vi "comm wait for character.vi"(5 "Loop Delay (10)":u32=10, 7 "timeout (10000)":u32=10000, 8 "error in (no error)":errorcluster, 9 "string in (\"\")":string, 10 "character":string, 11 "Comm Handle":u64) -> (0 "error out":errorcluster, 1 "received data":string, 2 "match":bool, 3 "dup Comm Handle":u64, 4 "before match":string, 6 "after match":string)   [LabVIEW 2021, in "lvserial.lvlib"]
doc: "This VI is receiving the data from the device and searches for the 'character'. If the character matches, the VI returns 'match'=TRUE.\nAfter 'timeout' the 'match' is FALSE and all received data are lost.\n\nThe VI receives only one byte at a time, so all data after the character remain in the serial I/O buffer."
uses:
  lvserial.lvlib
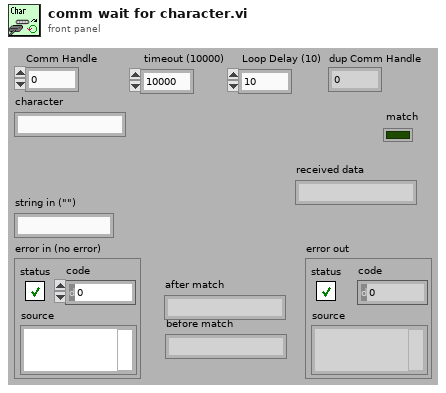
[diagram p1: front panel]
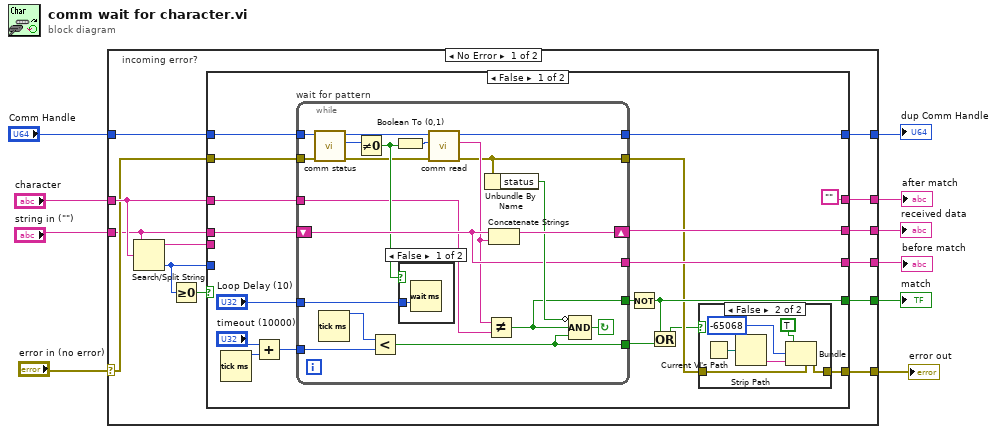
[diagram p0: block diagram]
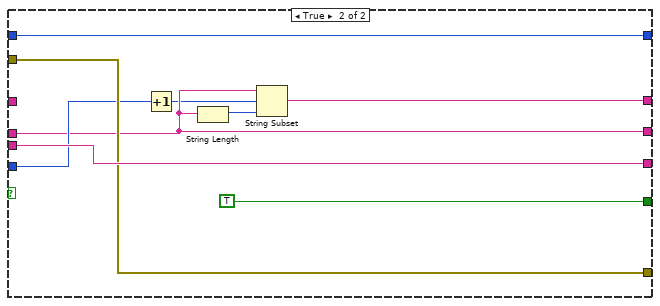
[diagram p4: hidden frame]
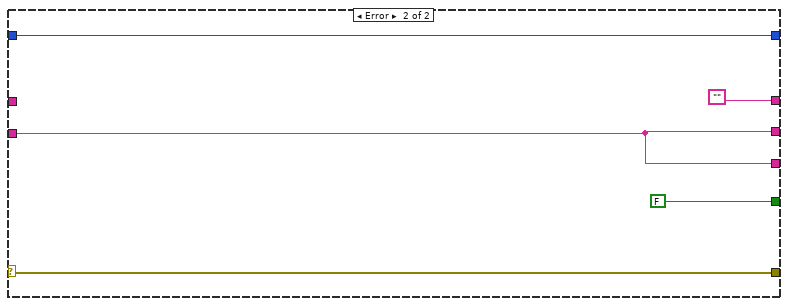
[diagram p5: hidden frame]
diagram:
  n1 = case "incoming error?" shown="No Error" "error in (no error)" {
    selector: "error in (no error)" -> [w12 w79]
    tunnel: [w23 FALSE] -> w10
    tunnel: [w20 w79] -> w1
    tunnel: "Comm Handle" -> [w22 w82]
    tunnel: [w21 w82] -> w8
    tunnel: [w19 w81] -> w7
    tunnel: [w18 w81] -> w6
    tunnel: "string in (\"\")" -> [w11 w81]
    tunnel: "character" -> [w17 _]
    tunnel: [w14 ""] -> w3
    frame No Error {
      n2 = Search/Split String(string=w11, search string/char (-)=w17) -> (substring before match=w15:string, offset of match=w13:i32)  [unwired: 2 out]
      n3 = Greater Or Equal To 0?(x=w13) -> (x >= 0?=w16:bool)
      n4 = case shown="False" w16 {
        tunnel: [w27 TRUE] -> w23
        tunnel: w22 -> [w40 w78]
        tunnel: [w37 w78] -> w21
        tunnel: [w26 w75] -> w20
        tunnel: w12 -> [w35 w75]
        tunnel: [w34 w71] -> w19
        tunnel: [w33 w77] -> w18
        tunnel: w17 -> [w32 _]
        tunnel: w11 -> [w31 w71]
        tunnel: w15 -> [_ w77]
        tunnel: ["" w73] -> w14
        tunnel: w13 -> [_ w74]
        frame False {
          n5 = Tick Count (ms)() -> (millisecond timer value=w39:u32)
          n6 = Add(x="timeout (10000)", y=w39) -> (x+y=w41:u32)
          n7 = while "wait for pattern" {
            tunnel: [w55] -> w33
            tunnel: [w49] -> w25
            tunnel: w35 -> [w46]
            tunnel: "Loop Delay (10)" -> [w53]
            tunnel: [w57] -> w29
            tunnel: [w48] -> w37
            tunnel: [w51] -> w28
            tunnel: w40 -> [w45]
            tunnel: w32 -> [w52]
            shift-left: w31 -> [w55]
            shift-right: [w59] -> w34
            tunnel: w41 -> [w60]
            stop <- w58 continue-if-true
            n8 = call "comm status.vi"("error in (no error)"=w46, "Comm Handle"=w45) -> ("error out"=w43:errorcluster, "In Queue"=w44:u32, "dup Comm Handle"=w42:u64)  [unwired: 7 out]
            n9 = Tick Count (ms)() -> (millisecond timer value=w61:u32)
            n10 = Not Equal To 0?(x=w44) -> (x != 0?=w54:bool)
            n11 = Less?(x=w61, y=w60) -> (x < y?=w57:bool)
            n12 = Boolean To (0,1)(Boolean=w54) -> (0, 1=w47:i16)
            n13 = case shown="False" w54 {
              tunnel: w53 -> [w62 _]
              frame False {
                n14 = Wait (ms)(milliseconds to wait=w62) -> ()  [unwired: 1 out]
              }
              frame True {
              }
            }
            n15 = call "comm read.vi"("error in (no error)"=w43, "requested byte count"=w47, "Comm Handle"=w42) -> ("error out"=w49:errorcluster, "string read"=w50:string, "dup Comm Handle"=w48:u64)  [unwired: 6 out]
            n16 = Unbundle By Name(w49) -> ("status"=w56:bool)
            n17 = Not Equal?(x=w50, y=w52) -> (x != y?=w51:bool)
            n18 = Concatenate Strings(w55, w50) -> (w59:string)
            n19 = Compound Arithmetic op=AND(invert w56, w51, w57) -> (w58:bool)
          }
          n20 = Not(x=w28) -> (.not. x?=w27:bool)
          n21 = Or(x=w27, y=w29) -> (x .or. y?=w24:bool)
          n22 = case shown="False" w24 {
            tunnel: w25 -> [w63 w69]
            tunnel: [w63 w68] -> w26
            frame True {
            }
            frame False {
              n23 = Current VI's Path() -> (path=w65:path)
              n24 = Strip Path(path=w65) -> (name=w66:string)  [unwired: 1 out]
              n25 = Bundle(cluster=w69, "status"=TRUE, "code"=-65068, "source"=w66) -> (w68:errorcluster)
            }
          }
        }
        frame True {
          n26 = Increment(x=w74) -> (x+1=w70:i32)
          n27 = String Length(string=w71) -> (length=w72:i32)
          n28 = String Subset(string=w71, offset (0)=w70, length (rest)=w72) -> (substring=w73:string)
        }
      }
    }
    frame Error {
    }
  }
  "match" <- w10
  "dup Comm Handle" <- w8
  "received data" <- w7
  "before match" <- w6
  "after match" <- w3
  "error out" <- w1
